vi "action.vi"(0 "HGF_FGV_VisitAll":refnum<class "HGF_FGV_VisitAll.lvclass">, 2 "Objects":refnum<class>[](array[class]), 5 "error in (no error)":errorcluster) -> (14 "dup HGF_FGV_VisitAll":refnum<class "HGF_FGV_VisitAll.lvclass">, 16 "dup Objects":refnum<class>[](array[class]), 19 "error out":errorcluster)   [LabVIEW 2012, in "HGF_FGV.lvlib" / "HGF_FGV_VisitAll.lvclass"]
doc: "Apply Visitors action to all objects in FGV instance."
uses:
  HGF_FGV_VisitAll.lvclass
  HGF_Visitable/HGF_Visitable.lvclass
  HGF_FGV_Visitor/HGF_FGV_Visitor.lvclass
  HGF_Visitor/HGF_Visitor.lvclass
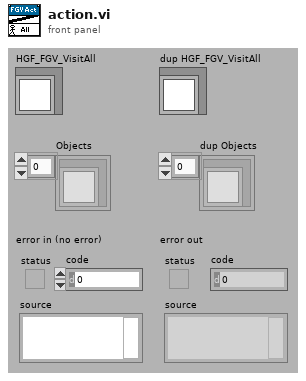
[diagram p1: front panel]
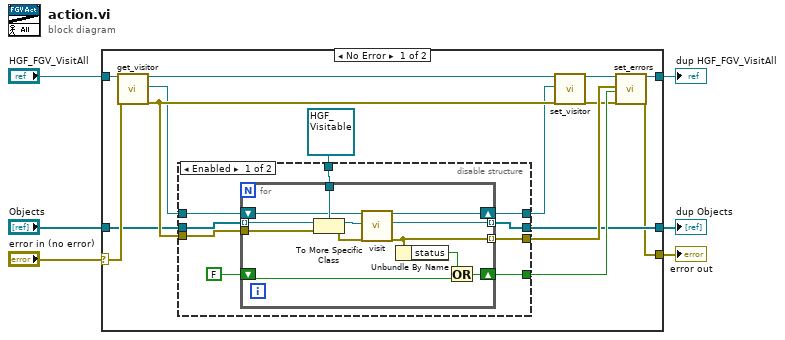
[diagram p0: block diagram]
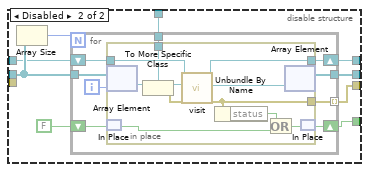
[diagram p2: hidden frame]
diagram:
  n1 = case shown="No Error" "error in (no error)" {
    selector: "error in (no error)" -> [w19 w74]
    tunnel: [w7 w74] -> w5
    tunnel: [w14 w73] -> w3
    tunnel: "HGF_FGV_VisitAll" -> [w21 w73]
    tunnel: [w10 w72] -> w2
    tunnel: "Objects" -> [w11 w72]
    frame No Error {
      n2 = call "get_visitor.vi"("HGF_FGV_Visitor"=w21, "error in (no error)"=w19) -> ("dup HGF_FGV_Visitor"=w20:refnum<class "HGF_FGV_VisitAll.lvclass">, "visitor"=w17:refnum<class "HGF_Visitor.lvclass">, "error out"=w18:errorcluster)  [unwired: 15 out]
      n3 = disable-structure shown="Enabled" {
        disable-tunnel: w18 -> [w30 _]
        disable-tunnel: w17 -> [w29 w46]
        disable-tunnel: [w28 w44] -> w16
        disable-tunnel: [w26 w43] -> w13
        disable-tunnel: [w25 w51] -> w12
        disable-tunnel: w11 -> [w24 w48]
        disable-tunnel: [w23 w47] -> w10
        disable-tunnel: refnum<class "HGF_Visitable.lvclass"> refnum ("HGF_Visitable.lvclass") -> [w22 w45]
        frame Enabled {
          n4 = for {
            tunnel: w24 -> [w42] mode=indexing
            tunnel: w22 -> [w41]
            tunnel: [w36] -> w23 mode=indexing
            shift-right: [w35] -> w28
            shift-left: w29 -> [w34]
            tunnel: w30 -> [w40]
            tunnel: [w31] -> w26 mode=indexing
            shift-right: [w39] -> w25
            shift-left: FALSE -> [w37]
            n5 = To More Specific Class(target class=w41, reference=w42, error in=w40) -> (specific class reference=w33:refnum<class "HGF_Visitable.lvclass">, error out=w32:errorcluster)
            n6 = call "visit.vi"("HGF_Visitor"=w34, "HGF_Visitable"=w33, "error in (no error)"=w32) -> ("dup HGF_Visitor"=w35:refnum<class "HGF_Visitor.lvclass">, "dup HGF_Visitable"=w36:refnum<class "HGF_Visitable.lvclass">, "error out"=w31:errorcluster)  [unwired: 14 out]
            n7 = Unbundle By Name(w31) -> ("status"=w38:bool)
            n8 = Or(x=w38, y=w37) -> (x .or. y?=w39:bool)
          }
        }
        frame Disabled {
          n9 = Array Size(array=w48) -> (size(s)=w49:i32)
          n10 = for {
            N: w49 -> [_]
            shift-right: [w54] -> w51
            shift-left: FALSE -> [w55]
            tunnel: w48 -> [w60]
            tunnel: [w58] -> w47
            tunnel: w45 -> [w56]
            shift-right: [w53] -> w44
            shift-left: w46 -> [w57]
            tunnel: [w52] -> w43 mode=indexing
            i -> [w59]
            n11 = in-place {
              in-place-border: w57 -> [w67]
              in-place-border: w56 -> [w66]
              in-place-border: [w62] -> w53
              in-place-border: [w61] -> w52
              n12 = in-place-array #1(w60, w59) -> (w68:refnum<class>)
              n13 = in-place-match #2(w55) -> (w65:bool)
              n14 = To More Specific Class(target class=w66, reference=w68) -> (specific class reference=w70:refnum<class "HGF_Visitable.lvclass">, error out=w69:errorcluster)  [unwired: 1 in]
              n15 = call "visit.vi"("HGF_Visitor"=w67, "HGF_Visitable"=w70, "error in (no error)"=w69) -> ("dup HGF_Visitor"=w62:refnum<class "HGF_Visitor.lvclass">, "dup HGF_Visitable"=w63:refnum<class "HGF_Visitable.lvclass">, "error out"=w61:errorcluster)  [unwired: 14 in]
              n16 = Unbundle By Name(w61) -> ("status"=w71:bool)
              n17 = Or(x=w71, y=w65) -> (x .or. y?=w64:bool)
              n18 = in-place-array #1(w63) -> (w58:refnum<class>[])  [unwired: 1 out]
              n19 = in-place-match #2(w64) -> (w54:bool)
            }
          }
        }
      }
      n20 = call "set_visitor.vi"("HGF_FGV_Visitor"=w20, "visitor"=w16, "error in (no error)"=w18) -> ("dup HGF_FGV_Visitor"=w15:refnum<class "HGF_FGV_VisitAll.lvclass">, "error out"=w8:errorcluster)  [unwired: 15 out]
      n21 = call "set_errors.vi"("HGF_FGV_Visitor"=w15, "Errors"=w13, "error"=w12, "error in (no error)"=w8) -> ("dup HGF_FGV_Visitor"=w14:refnum<class "HGF_FGV_VisitAll.lvclass">, "error out"=w7:errorcluster)  [unwired: 14 out]
    }
    frame Error {
    }
  }
  "error out" <- w5
  "dup HGF_FGV_VisitAll" <- w3
  "dup Objects" <- w2
